vi "xijk_create_search_list.vi"(7 "file path cluster in":T2, 8 "error in":errorcluster, 9 "correct paths?":bool=TRUE, 10 "queue in":refnum<queue>, 11 "search paths in":T1={"Paths"={"Path: Excitation filters"=path "", "Path: Dicroic filters"=path "", "Path: Emission filters"=path "", "Path reget"=path ""}, "table excitation"=[], "table dicroics"=[], "table emission"=[], "Integers"={"Select result n°"=1}, "boolean selector array"=[], "table for calculation automagic"=[]}) -> (0 "error out":errorcluster, 2 "queue out":refnum<queue>, 5 "search paths out":T1={"Paths"={"Path: Excitation filters"=path "", "Path: Dicroic filters"=path "", "Path: Emission filters"=path "", "Path reget"=path ""}, "table excitation"=[], "table dicroics"=[], "table emission"=[], "Integers"={"Select result n°"=1}, "boolean selector array"=[], "table for calculation automagic"=[]})   [LabVIEW 2010]
uses:
  Type Def/filepath.ctl
  Type Def/search_parameters.ctl
  <vilib>/Utility/file.llb/Write To Spreadsheet File (string).vi
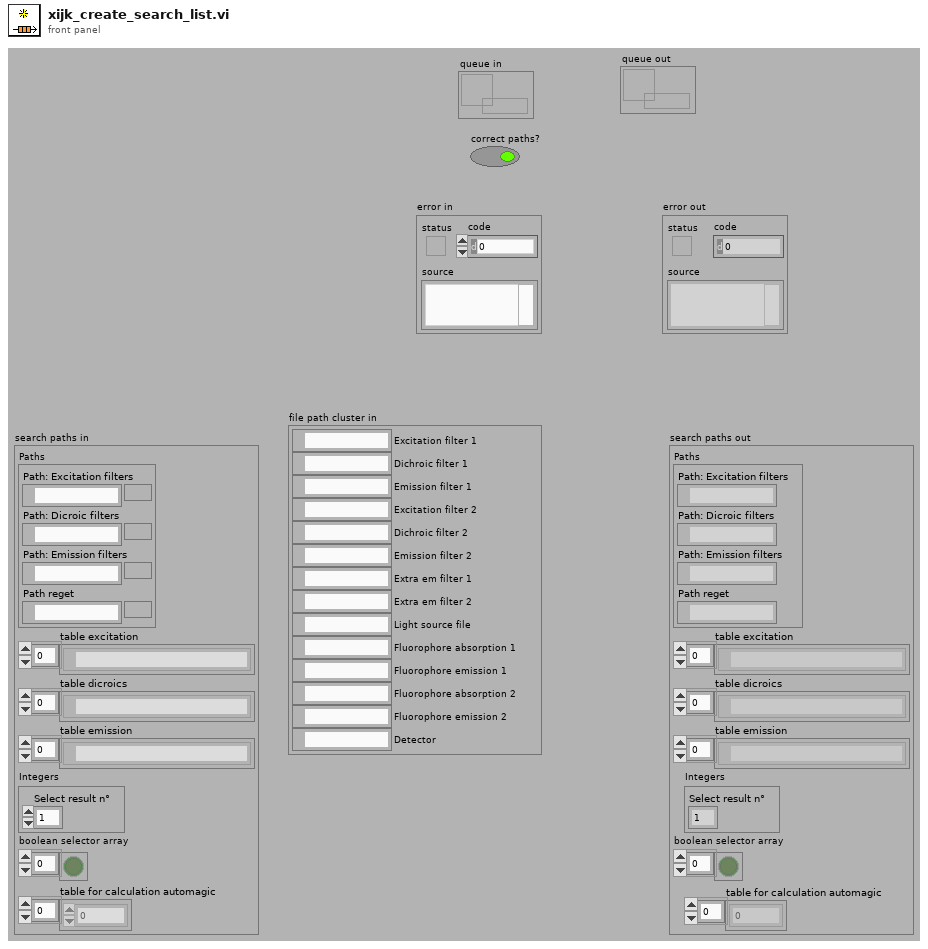
[diagram p1: front panel]
types:
  T1 = typedef "search_parameters.ctl" = cluster{"Paths":cluster{"Path: Excitation filters":path, "Path: Dicroic filters":path, "Path: Emission filters":path, "Path reget":path}, "table excitation":path[], "table dicroics":path[], "table emission":path[], "Integers":cluster{"Select result n°":u32}, "boolean selector array":bool[], "table for calculation automagic":i32[]}
  T2 = typedef "filepath.ctl" = cluster{"Excitation filter 1":path, "Dichroic filter 1":path, "Emission filter 1":path, "Excitation filter 2":path, "Dichroic filter 2":path, "Emission filter 2":path, "Extra em filter 1":path, "Extra em filter 2":path, "Light source file":path, "Fluorophore absorption 1":path, "Fluorophore emission 1":path, "Fluorophore absorption 2":path, "Fluorophore emission 2":path, "Detector":path}
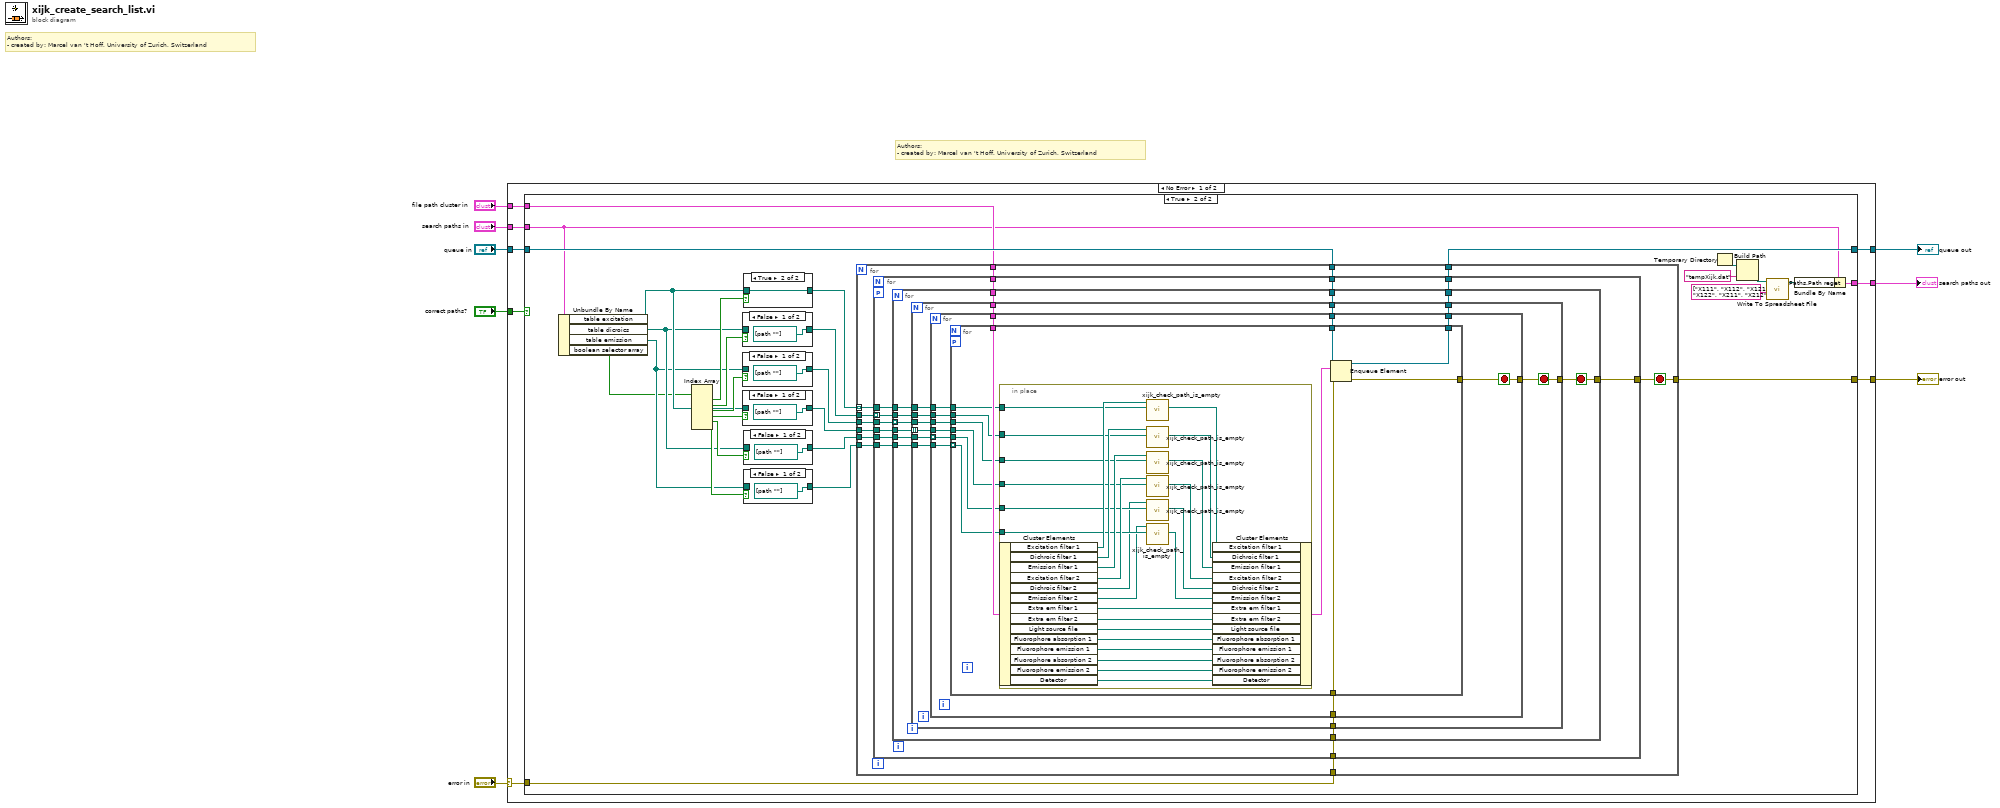
[diagram p0: block diagram]
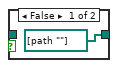
[diagram p8: hidden frame]
diagram:
  # "Authors: \n- created by: Marcel van 't Hoff, University of Zurich, Switzerland"
  # "Authors: \n- created by: Marcel van 't Hoff, University of Zurich, Switzerland"
  n1 = case shown="No Error" "error in" {
    selector: "error in" -> [w15 w155]
    tunnel: [w13 w154] -> w2
    tunnel: [w16 w155] -> w8
    tunnel: "queue in" -> [w14 w154]
    tunnel: "file path cluster in" -> [w12 _]
    tunnel: "search paths in" -> [w11 w153]
    tunnel: [w9 w153] -> w4
    tunnel: "correct paths?" -> [w10 _]
    frame No Error {
      n2 = case shown="True" w10 {
        tunnel: [w17 w20] -> w16
        tunnel: w15 -> [w17 w35]
        tunnel: w14 -> [w19 w34]
        tunnel: [w19 w33] -> w13
        tunnel: w12 -> [_ w32]
        tunnel: w11 -> [w18 w25]
        tunnel: [w18 w24] -> w9
        frame False {
        }
        frame True {
          n3 = Unbundle By Name(w25) -> ("table excitation"=w31:path[], "table dicroics"=w30:path[], "table emission"=w29:path[], "boolean selector array"=w28:bool[])
          n4 = Index Array(array=w28) -> (element #1=w47:bool, element #2=w40:bool, element #3=w39:bool, element #4=w38:bool, element #5=w37:bool, element #6=w36:bool)  [unwired: 6 in]
          n5 = case shown="False" w40 {
            tunnel: [path[] [path ""] ("table excitation") w57] -> w45
            tunnel: w30 -> [_ w57]
            frame False {
            }
            frame True {
            }
          }
          n6 = case shown="False" w39 {
            tunnel: [path[] [path ""] ("table excitation") w55] -> w44
            tunnel: w29 -> [_ w55]
            frame False {
            }
            frame True {
            }
          }
          n7 = case shown="False" w38 {
            tunnel: [path[] [path ""] ("table excitation") w53] -> w43
            tunnel: w31 -> [_ w53]
            frame False {
            }
            frame True {
            }
          }
          n8 = case shown="True" w47 {
            tunnel: w31 -> [_ w152]
            tunnel: [path[] [path ""] ("table excitation") w152] -> w46
            frame False {
            }
            frame True {
            }
          }
          n9 = case shown="False" w37 {
            tunnel: [path[] [path ""] ("table excitation") w51] -> w42
            tunnel: w30 -> [_ w51]
            frame False {
            }
            frame True {
            }
          }
          n10 = case shown="False" w36 {
            tunnel: [path[] [path ""] ("table excitation") w49] -> w41
            tunnel: w29 -> [_ w49]
            frame False {
            }
            frame True {
            }
          }
          n11 = for {
            tunnel: w44 -> [w68]
            tunnel: w45 -> [w67]
            tunnel: w46 -> [w66] mode=indexing
            tunnel: w43 -> [w65]
            tunnel: w42 -> [w64]
            tunnel: w41 -> [w63]
            tunnel: [w62] -> w33
            tunnel: w34 -> [w61]
            tunnel: [w58] -> w20
            tunnel: w35 -> [w60]
            tunnel: w32 -> [w59]
            stop <- w58 stop-if-true
            n12 = for {
              tunnel: w68 -> [w79]
              tunnel: w67 -> [w78] mode=indexing
              tunnel: w66 -> [w77]
              tunnel: w65 -> [w76]
              tunnel: w64 -> [w75]
              tunnel: w63 -> [w74]
              tunnel: [w73] -> w62
              tunnel: w61 -> [w72]
              tunnel: [w69] -> w58
              tunnel: w60 -> [w71]
              tunnel: w59 -> [w70]
              workers-P: _ -> [_]
              n13 = for {
                tunnel: w79 -> [w90] mode=indexing
                tunnel: w78 -> [w89]
                tunnel: w77 -> [w88]
                tunnel: w76 -> [w87]
                tunnel: w75 -> [w86]
                tunnel: w74 -> [w85]
                tunnel: [w84] -> w73
                tunnel: w72 -> [w83]
                tunnel: [w80] -> w69
                tunnel: w71 -> [w82]
                tunnel: w70 -> [w81]
                stop <- w80 stop-if-true
                n14 = for {
                  tunnel: w90 -> [w101]
                  tunnel: w89 -> [w100]
                  tunnel: w88 -> [w99]
                  tunnel: w87 -> [w98] mode=indexing
                  tunnel: w86 -> [w97]
                  tunnel: w85 -> [w96]
                  tunnel: [w95] -> w84
                  tunnel: w83 -> [w94]
                  tunnel: [w91] -> w80
                  tunnel: w82 -> [w93]
                  tunnel: w81 -> [w92]
                  stop <- w91 stop-if-true
                  n15 = for {
                    tunnel: w101 -> [w112]
                    tunnel: w100 -> [w111]
                    tunnel: w99 -> [w110]
                    tunnel: w98 -> [w109]
                    tunnel: w97 -> [w108] mode=indexing
                    tunnel: w96 -> [w107]
                    tunnel: [w106] -> w95
                    tunnel: w94 -> [w105]
                    tunnel: [w102] -> w91
                    tunnel: w93 -> [w104]
                    tunnel: w92 -> [w103]
                    stop <- w102 stop-if-true
                    n16 = for {
                      tunnel: w112 -> [w118]
                      tunnel: w111 -> [w119]
                      tunnel: w110 -> [w120]
                      tunnel: w109 -> [w117]
                      tunnel: w108 -> [w116]
                      tunnel: w107 -> [w115] mode=indexing
                      tunnel: [w124] -> w106
                      tunnel: w105 -> [w123]
                      tunnel: [w113] -> w102
                      tunnel: w104 -> [w122]
                      tunnel: w103 -> [w121]
                      workers-P: _ -> [_]
                      n17 = in-place {
                        in-place-border: w120 -> [w149]
                        in-place-border: w119 -> [w146]
                        in-place-border: w118 -> [w144]
                        in-place-border: w117 -> [w142]
                        in-place-border: w116 -> [w141]
                        in-place-border: w115 -> [w140]
                        n18 = in-place-cluster #1(w121) -> ("Excitation filter 1"=w150:path, "Dichroic filter 1"=w147:path, "Emission filter 1"=w145:path, "Excitation filter 2"=w143:path, "Dichroic filter 2"=w139:path, "Emission filter 2"=w138:path, "Extra em filter 1"=w132:path, "Extra em filter 2"=w131:path, "Light source file"=w130:path, "Fluorophore absorption 1"=w129:path, "Fluorophore emission 1"=w128:path, "Fluorophore absorption 2"=w127:path, "Fluorophore emission 2"=w126:path, "Detector"=w125:path)
                        n19 = call "xijk_check_path_is_empty.vi"("Excitation filter 2"=w149, "Path"=w150) -> ("Excitation filter 1"=w148:path)  [unwired: 9 in]
                        n20 = call "xijk_check_path_is_empty.vi"("Excitation filter 2"=w146, "Path"=w147) -> ("Excitation filter 1"=w137:path)  [unwired: 9 in]
                        n21 = call "xijk_check_path_is_empty.vi"("Excitation filter 2"=w144, "Path"=w145) -> ("Excitation filter 1"=w136:path)  [unwired: 9 in]
                        n22 = call "xijk_check_path_is_empty.vi"("Excitation filter 2"=w142, "Path"=w143) -> ("Excitation filter 1"=w135:path)  [unwired: 9 in]
                        n23 = call "xijk_check_path_is_empty.vi"("Excitation filter 2"=w141, "Path"=w139) -> ("Excitation filter 1"=w134:path)  [unwired: 9 in]
                        n24 = call "xijk_check_path_is_empty.vi"("Excitation filter 2"=w140, "Path"=w138) -> ("Excitation filter 1"=w133:path)  [unwired: 9 in]
                        n25 = in-place-cluster #1("Excitation filter 1"=w148, "Dichroic filter 1"=w137, "Emission filter 1"=w136, "Excitation filter 2"=w135, "Dichroic filter 2"=w134, "Emission filter 2"=w133, "Extra em filter 1"=w132, "Extra em filter 2"=w131, "Light source file"=w130, "Fluorophore absorption 1"=w129, "Fluorophore emission 1"=w128, "Fluorophore absorption 2"=w127, "Fluorophore emission 2"=w126, "Detector"=w125) -> (w114:T2)
                      }
                      n26 = Enqueue Element(queue=w123, element=w114, error in (no error)=w122) -> (queue out=w124:refnum<queue>, error out=w113:errorcluster)  [unwired: 1 in, 1 out]
                    }
                  }
                }
              }
            }
          }
          n27 = Temporary Directory() -> (w22:path)
          n28 = Build Path(base path=w22, name or relative path="tempXijk.dat") -> (appended path=w21:path)
          n29 = call-poly <vilib>:"Write To Spreadsheet File.vi"("1D data"=string[] ["X111", "X112", "X121", "X122", "X211", "X212", "X221", "X222", "E111", "E112", "E121", "E122", "E211", "E212", "E221", "E222", "EX1", "DIC1", "EM1", "EX2", "DIC2", "EM2"], "file path (dialog if empty)"=w21) -> ("new file path (Not A Path if cancelled)"=w27:path)  [unwired: 4 in, 2 out]
          n30 = Bundle By Name(cluster=w25, "Paths.Path reget"=w27) -> (w24:T1)
        }
      }
    }
    frame Error {
    }
  }
  "error out" <- w8
  "search paths out" <- w4
  "queue out" <- w2
